vi "producer.vi"() -> ()   [LabVIEW 2015]
panel:
  in  "Numeric":u32=5000
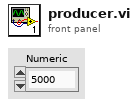
[diagram p1: front panel]
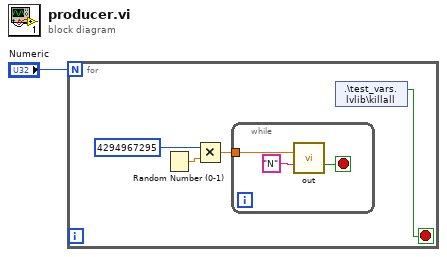
[diagram p0: block diagram]
diagram:
  n1 = for {
    N: "Numeric" -> [_]
    stop <- w2 stop-if-true
    n2 = Random Number (0-1)() -> (number: 0 to 1=w3:dbl)
    n3 = Multiply(x=u32 4294967295, y=w3) -> (x*y=w4:dbl)
    n4 = while {
      tunnel: w4 -> [w8]
      stop <- w6 stop-if-true
      n5 = call "out.vi"("IN VARIANT"=w8, "Name in"="N") -> ("Operation Ok"=w6:bool)  [unwired: 12 in, 1 out]
    }
    n6 = shared-variable ".\\test_vars.lvlib\\killall"() -> (w2:bool)  [unwired: 1 in, 1 out]
  }
